vi "FdxCmdEDESubCreateCvi.vi"(8 "error in":errorcluster, 9 "OwnSubscriberIndex":u32, 11 "InstrumentHandle":u32) -> (0 "error out":errorcluster, 2 "EDESubscriberHandle":u32, 3 "InstrumentHandle":u32)   [LabVIEW 2020, in "AIM664LV.lvlib"]
doc: "This function is used to create and configure the communication parameters needed to\nsimulate an EDE Subscriber."
uses:
  AIM664LV.lvlib
  AFDX_LibraryAdmin/FdxGlobalDllPath.vi
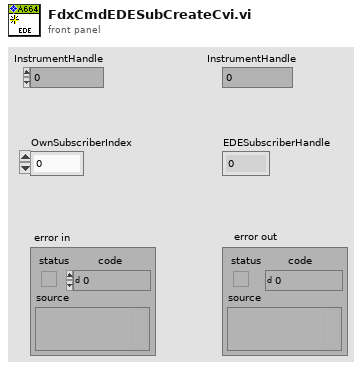
[diagram p1: front panel]
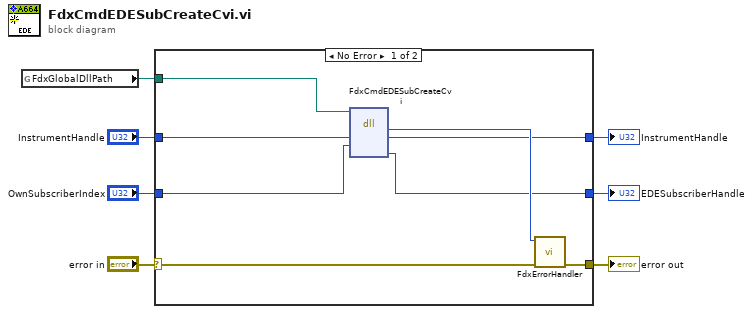
[diagram p0: block diagram]
diagram:
  n1 = global read "FdxGlobalDllPath.vi" "FdxGlobalDllPath"() -> (w5:path)
  n2 = case shown="No Error" "error in" {
    selector: "error in" -> [w14 w17]
    tunnel: [w15 w17] -> w7
    tunnel: w5 -> [w12 _]
    tunnel: "InstrumentHandle" -> [w11 w16]
    tunnel: "OwnSubscriberIndex" -> [w10 _]
    tunnel: [w9 w16] -> w2
    tunnel: [w8 _] -> w1
    frame No Error {
      n3 = dll-call lib="aim_fdx.19.dll" fn="FdxCmdEDESubCreateCvi"(path in=w12, "InstrumentHandle"=w11, "OwnSubscriberIndex"=w10) -> ("status"=w13:i32, "InstrumentHandle"=w9:u32, "EDESubscriberHandle"=w8:u32)  [unwired: 3 in, 3 out]
      n4 = call "FdxErrorHandler.vi"("error in"=w14, "AIM Error"=w13) -> ("error out"=w15:errorcluster)  [unwired: 9 in]
    }
    frame Error {
    }
  }
  "error out" <- w7
  "InstrumentHandle" <- w2
  "EDESubscriberHandle" <- w1
